vi "Launch API Tester.vi"(8 "error in":errorcluster, 11 "VI in":refnum<vi>) -> (0 "error out":errorcluster)   [LabVIEW 2020, in "Launcher Support.lvlib"]
uses:
  Launcher Support.lvlib
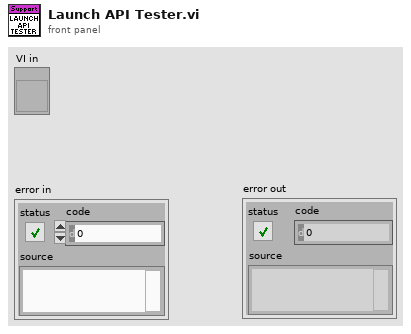
[diagram p1: front panel]
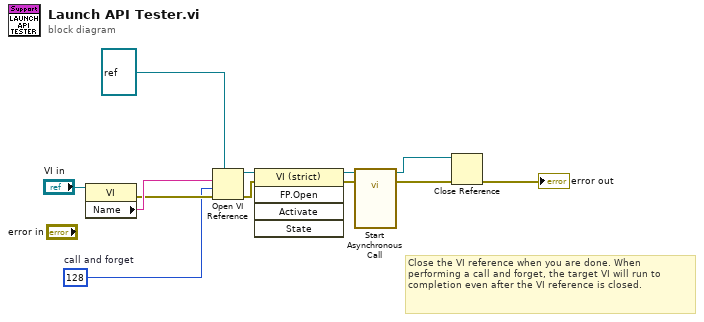
[diagram p0: block diagram]
diagram:
  w5 = 128  # call and forget
  # "Close the VI reference when you are done. When performing a call and forget, the target VI will run to completion even after the VI reference is closed."
  n1 = property class="VI"(reference="VI in") -> (error out=w6:errorcluster, "Name"=w7:string)  [unwired: 1 in, 1 out]
  n2 = Open VI Reference(type specifier VI Refnum (for type only)=refnum<vi> refnum, vi path=w7, options=w5, error in (no error)=w6) -> (vi reference=w12:refnum<vi>, error out=w4:errorcluster)  [unwired: 2 in]
  n3 = invoke class="VI (strict)" method="FP.Open"(reference=w12, error in=w4) -> (reference out=w11:refnum<vi>, error out=w3:errorcluster)  [unwired: 3 in, 3 out]
  n4 = call-by-ref "Start Asynchronous Call"(reference=w11, error in=w3) -> (reference out=w9:refnum<vi>, error out=w2:errorcluster)  [unwired: 12 in]
  n5 = Close Reference(reference=w9, error in (no error)=w2) -> (error out=→"error out":errorcluster)
